vi "Dispose & Teminate.vi"(0 "DBMap in":refnum<class "DBMap.lvclass">, 11 "error in (no error)":errorcluster {"code" format="Error %.0f"}) -> (4 "DBMap out":refnum<class "DBMap.lvclass">, 15 "error out":errorcluster {"code" format="Error %.0f"})   [LabVIEW 2024, in "DBMap.lvclass"]
uses:
  DBMap.lvclass
  DBMap.lvclass/DBMap.ctl
  <vilib>/drjdpowell/SQLite Library/SQL Connection/Connection.lvclass
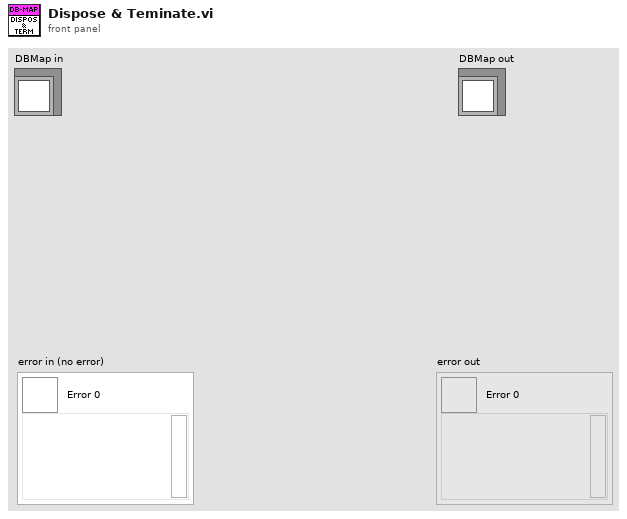
[diagram p1: front panel]
types:
  T1 = typedef "Semaphore RefNum" = refnum<k1>
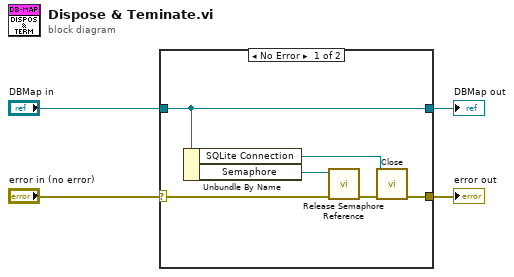
[diagram p0: block diagram]
diagram:
  n1 = case shown="No Error" "error in (no error)" {
    selector: "error in (no error)" -> [w7 w12]
    tunnel: [w8 w12] -> w3
    tunnel: [w10 w11] -> w1
    tunnel: "DBMap in" -> [w10 w11]
    frame No Error {
      n2 = Unbundle By Name(w10) -> ("SQLite Connection"=w9:refnum<class "Connection.lvclass">, "Semaphore"=w5:T1)
      n3 = call <vilib>:"Release Semaphore Reference.vi"("error in (no error)"=w7, "semaphore"=w5) -> ("error out"=w6:errorcluster)  [unwired: 8 in, 1 out]
      n4 = call-dynamic "Close.vi"("error in (no error)"=w6, "SQLite Connection in"=w9) -> ("error out"=w8:errorcluster)  [unwired: 9 in]
    }
    frame Error {
    }
  }
  "error out" <- w3
  "DBMap out" <- w1
